vi "BSONElementProbe.vi"(11 "response":refnum<class "tBSONElement.lvclass">) -> (2 "Value":string, 3 "Boolean":bool)   [LabVIEW 2013, in "BSON.lvlib" / "tBSONElement.lvclass"]
uses:
  tBSONElement.lvclass
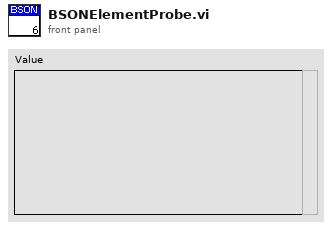
[diagram p1: front panel]
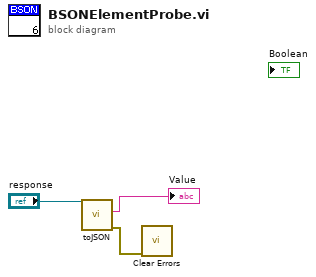
[diagram p0: block diagram]
diagram:
  n1 = call-dynamic "toJSON.vi"("tBSONElement in"="response") -> ("error out"=w2:errorcluster, "JSON"=→"Value":string)  [unwired: 8 in, 1 out]
  n2 = call <vilib>:"Clear Errors.vi"("error in (no error)"=w2) -> ()  [unwired: 6 in, 1 out]
